vi "set ring control values.vi"(8 "error in (no error)":errorcluster, 10 "config data":T1, 11 "Ring Ref":refnum<vi>[](array[refnum])) -> (0 "error out":errorcluster)   [LabVIEW 2024, in "Ring Control Management.lvlib"]
doc: "This VI dynamically sets each control referenced in <b>Ring Ref</b> to a specific item defined by the <b>config data</b> cluster at runtime.\n\nThe <b>config data</b> cluster contains a 2-D array with section names and the number of keys they contain, a 1-D array with key names (not used in this VI), and another 1-D array with key values, which are used as the item names for the Ring controls."
uses:
  Ring Control Management.lvlib
  config data.ctl
  API Config Files Management.lvlib
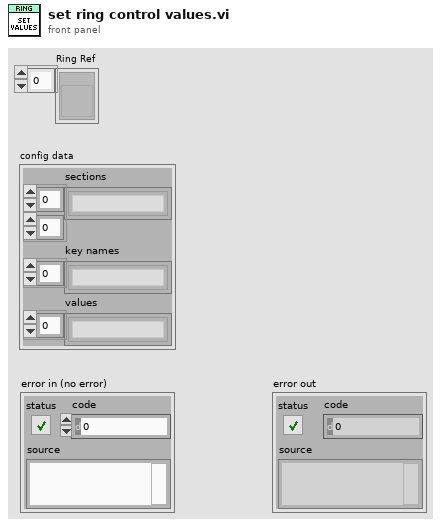
[diagram p1: front panel]
types:
  T1 = typedef "API Config Files Management.lvlib/config data.ctl" = cluster{"sections":string[][], "key names":string[], "values":string[]}
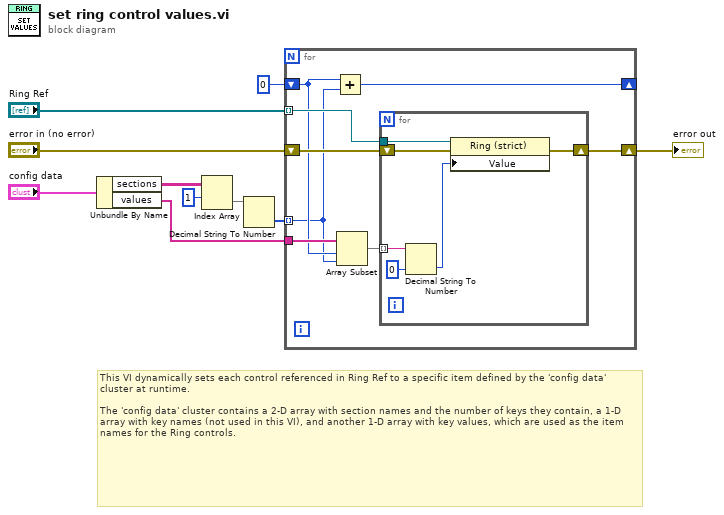
[diagram p0: block diagram]
diagram:
  # "This VI dynamically sets each control referenced in Ring Ref to a specific item defined by the 'config data' cluster at runtime.\n\nThe 'config data' cluster contains a 2-D array with section names and the number of keys they contain, a 1-D array with key names (not used in this VI), and another 1-D array with key values, which are used as the item names for the Ring controls."
  n1 = Unbundle By Name("config data") -> ("sections"=w2:string[][], "values"=w1:string[])
  n2 = Index Array(array=w2, index (row)=1) -> (element=w4:string[])  [unwired: 1 in]
  n3 = Decimal String To Number(string=w4) -> (number=w5:i32[])  [unwired: 2 in, 1 out]
  n4 = for {
    tunnel: "Ring Ref" -> [w18] mode=indexing
    shift-right: [w16] -> w10
    shift-left: "error in (no error)" -> [w17]
    tunnel: w5 -> [w12] mode=indexing
    tunnel: w1 -> [w14]
    shift-right: [w15] -> _
    shift-left: 0 -> [w13]
    n5 = Add(x=w13, y=w12) -> (x+y=w15:i32)
    n6 = Array Subset(array=w14, index=w13, length=w12) -> (w11:string[])
    n7 = for {
      tunnel: w18 -> [w24]
      tunnel: w11 -> [w22] mode=indexing
      shift-right: [w19] -> w16
      shift-left: w17 -> [w23]
      n8 = Decimal String To Number(string=w22, default (0L)=u16 0 ("default (0 I32)")) -> (number=w20:u16)  [unwired: 1 in, 1 out]
      n9 = property on="Property Node" class="Ring (strict)"(reference=w24, error in=w23, "Value"=w20) -> (error out=w19:errorcluster)  [unwired: 1 out]
    }
  }
  "error out" <- w10
